vi "RichToFlatgoogle_protobuf_Enum.vi"(5 "OutputClusterType":T1, 11 "InputCluster":T7) -> (3 "OutputCluster":T1)   [LabVIEW 2021, in "ni.measurementlink.measurement.v1.api.lvlib"]
uses:
  ni.measurementlink.measurement.v1.api.lvlib
  google_protobuf_Enum.ctl
  google_protobuf_EnumValue.ctl
  google_protobuf_Option.ctl
  google_protobuf_Any.ctl
  google_protobuf_SourceContext.ctl
  google_protobuf_Syntax.ctl
  google_protobuf_Enum_Flat.ctl
  google_protobuf_EnumValue_Flat.ctl
  google_protobuf_Option_Flat.ctl
  google_protobuf_Any_Flat.ctl
  google_protobuf_SourceContext_Flat.ctl
  RichToFlatgoogle_protobuf_Any.vi
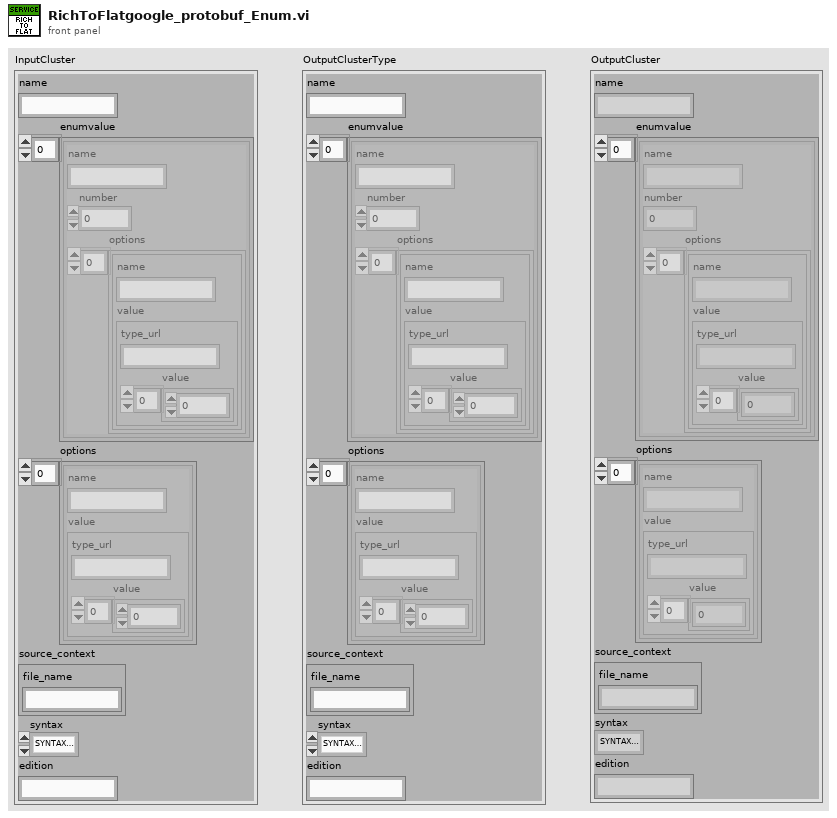
[diagram p1: front panel]
types:
  T1 = typedef "ni.measurementlink.measurement.v1.api.lvlib/google_protobuf_Enum_Flat.ctl" = cluster{"name":string, "enumvalue":T2[], "options":T3[], "source_context":T5, "syntax":T6, "edition":string}
  T2 = typedef "ni.measurementlink.measurement.v1.api.lvlib/google_protobuf_EnumValue_Flat.ctl" = cluster{"name":string, "number":i32, "options":T3[]}
  T3 = typedef "ni.measurementlink.measurement.v1.api.lvlib/google_protobuf_Option_Flat.ctl" = cluster{"name":string, "value":T4}
  T4 = typedef "ni.measurementlink.measurement.v1.api.lvlib/google_protobuf_Any_Flat.ctl" = cluster{"type_url":string, "value":u8[]}
  T5 = typedef "ni.measurementlink.measurement.v1.api.lvlib/google_protobuf_SourceContext_Flat.ctl" = cluster{"file_name":string}
  T6 = typedef "ni.measurementlink.measurement.v1.api.lvlib/google_protobuf_Syntax.ctl" = enum32{"SYNTAX_PROTO2", "SYNTAX_PROTO3", "SYNTAX_EDITIONS"}
  T7 = typedef "ni.measurementlink.measurement.v1.api.lvlib/google_protobuf_Enum.ctl" = cluster{"name":string, "enumvalue":T8[], "options":T9[], "source_context":T11, "syntax":T6, "edition":string}
  T8 = typedef "ni.measurementlink.measurement.v1.api.lvlib/google_protobuf_EnumValue.ctl" = cluster{"name":string, "number":i32, "options":T9[]}
  T9 = typedef "ni.measurementlink.measurement.v1.api.lvlib/google_protobuf_Option.ctl" = cluster{"name":string, "value":T10}
  T10 = typedef "ni.measurementlink.measurement.v1.api.lvlib/google_protobuf_Any.ctl" = cluster{"type_url":string, "value":u8[]}
  T11 = typedef "ni.measurementlink.measurement.v1.api.lvlib/google_protobuf_SourceContext.ctl" = cluster{"file_name":string}
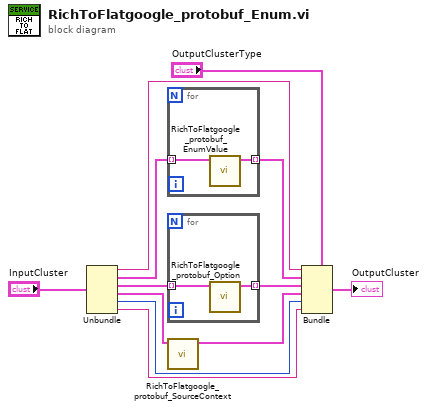
[diagram p0: block diagram]
diagram:
  n1 = Unbundle "Unbundle"("InputCluster") -> ("name"=w9:string, "enumvalue"=w8:T8[], "options"=w6:T9[], "source_context"=w4:T11, "syntax"=w2:T6, "edition"=w1:string)
  n2 = for {
    tunnel: w8 -> [w14] mode=indexing
    tunnel: [w13] -> w7 mode=indexing
    n3 = call "RichToFlatgoogle_protobuf_EnumValue.vi"("InputCluster"=w14) -> ("OutputCluster"=w13:T2)  [unwired: 10 in]
  }
  n4 = for {
    tunnel: w6 -> [w16] mode=indexing
    tunnel: [w15] -> w5 mode=indexing
    n5 = call "RichToFlatgoogle_protobuf_Option.vi"("InputCluster"=w16) -> ("OutputCluster"=w15:T3)  [unwired: 10 in]
  }
  n6 = call "RichToFlatgoogle_protobuf_SourceContext.vi"("InputCluster"=w4) -> ("OutputCluster"=w3:T5)  [unwired: 10 in]
  n7 = Bundle "Bundle"(cluster="OutputClusterType", "name"=w9, "enumvalue"=w7, "options"=w5, "source_context"=w3, "syntax"=w2, "edition"=w1) -> (→"OutputCluster":T1)
